vi "Set Lockin Oscillator.vi"(7 "Model":enum16{"7265", "SR830"}(ring)=enum."SR830", 9 "Amplitude":dbl=-1.0, 10 "Frequency":dbl=-1.0, 11 "VISA resource name":refnum<visa-resource-name>) -> (1 "Actual Amp":dbl, 2 "Actual Freq":dbl)   [LabVIEW 2021]
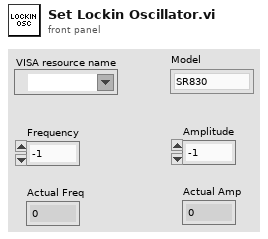
[diagram p1: front panel]
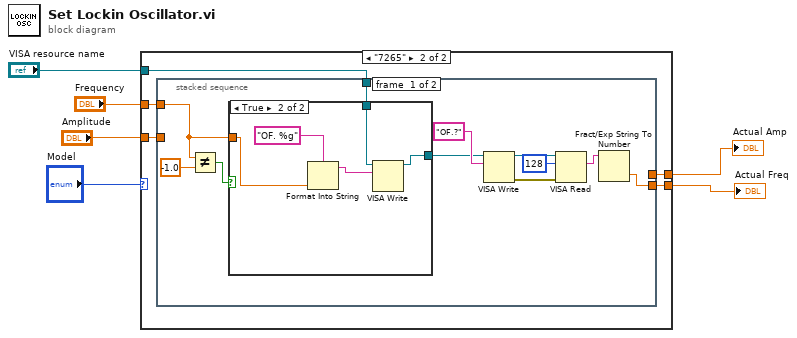
[diagram p0: block diagram]
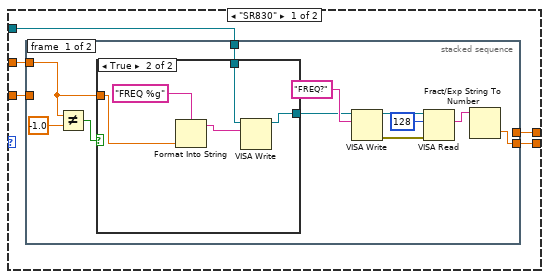
[diagram p2: hidden frame]
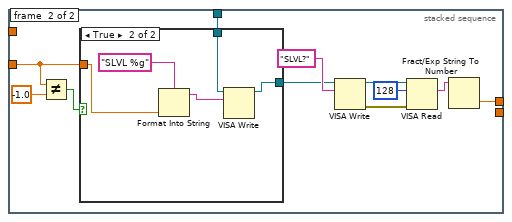
[diagram p4: hidden frame]
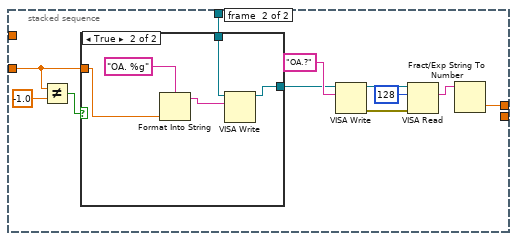
[diagram p7: hidden frame]
diagram:
  n1 = case shown="\"7265\"" "Model" {
    tunnel: "Frequency" -> [w11 w50]
    tunnel: "VISA resource name" -> [w10 w49]
    tunnel: [w9 w48] -> w3
    tunnel: "Amplitude" -> [w7 w47]
    tunnel: [w8 w46] -> w1
    frame "SR830" {
      n2 = stacked-sequence {
        tunnel: w11 -> [w20 _]
        tunnel: w10 -> [w19 w37]
        tunnel: [w12 _] -> w9
        tunnel: [_ w30] -> w8
        tunnel: w7 -> [_ w29]
        frame #0 {
          n3 = Not Equal?(x=w20, y=-1.0) -> (x != y?=w22:bool)
          n4 = case shown="True" w22 {
            tunnel: w20 -> [_ w27]
            tunnel: w19 -> [w23 w25]
            tunnel: [w23 w24] -> w13
            frame False {
            }
            frame True {
              n5 = Format Into String(format string="FREQ %g", w27) -> (resulting string=w26:string)  [unwired: 2 in, 1 out]
              n6 = VISA Write(VISA resource name=w25, write buffer=w26) -> (VISA resource name out=w24:refnum<visa-resource-name>)  [unwired: 1 in, 2 out]
            }
          }
          n7 = VISA Write(VISA resource name=w13, write buffer="FREQ?" ("format string")) -> (VISA resource name out=w17:refnum<visa-resource-name>, error out=w15:errorcluster)  [unwired: 1 in, 1 out]
          n8 = VISA Read(VISA resource name=w17, byte count=u32 128, error in (no error)=w15) -> (read buffer=w14:string)  [unwired: 3 out]
          n9 = Fract/Exp String To Number(string=w14) -> (number=w12:dbl)  [unwired: 3 in, 1 out]
        }
        frame #1 {
          n10 = Not Equal?(x=w29, y=-1.0) -> (x != y?=w39:bool)
          n11 = case shown="True" w39 {
            tunnel: w29 -> [_ w44]
            tunnel: w37 -> [w40 w42]
            tunnel: [w40 w41] -> w31
            frame False {
            }
            frame True {
              n12 = Format Into String(format string="SLVL %g", w44) -> (resulting string=w43:string)  [unwired: 2 in, 1 out]
              n13 = VISA Write(VISA resource name=w42, write buffer=w43) -> (VISA resource name out=w41:refnum<visa-resource-name>)  [unwired: 1 in, 2 out]
            }
          }
          n14 = VISA Write(VISA resource name=w31, write buffer="SLVL?" ("format string")) -> (VISA resource name out=w35:refnum<visa-resource-name>, error out=w33:errorcluster)  [unwired: 1 in, 1 out]
          n15 = VISA Read(VISA resource name=w35, byte count=u32 128, error in (no error)=w33) -> (read buffer=w32:string)  [unwired: 3 out]
          n16 = Fract/Exp String To Number(string=w32) -> (number=w30:dbl)  [unwired: 3 in, 1 out]
        }
      }
    }
    frame "7265" {
      n17 = stacked-sequence {
        tunnel: w50 -> [w59 _]
        tunnel: w49 -> [w58 w76]
        tunnel: [w51 _] -> w48
        tunnel: w47 -> [_ w69]
        tunnel: [_ w68] -> w46
        frame #0 {
          n18 = Not Equal?(x=w59, y=-1.0) -> (x != y?=w61:bool)
          n19 = case shown="True" w61 {
            tunnel: w59 -> [_ w66]
            tunnel: w58 -> [w62 w64]
            tunnel: [w62 w63] -> w52
            frame False {
            }
            frame True {
              n20 = Format Into String(format string="OF. %g", w66) -> (resulting string=w65:string)  [unwired: 2 in, 1 out]
              n21 = VISA Write(VISA resource name=w64, write buffer=w65) -> (VISA resource name out=w63:refnum<visa-resource-name>)  [unwired: 1 in, 2 out]
            }
          }
          n22 = VISA Write(VISA resource name=w52, write buffer="OF.?" ("format string")) -> (VISA resource name out=w56:refnum<visa-resource-name>, error out=w54:errorcluster)  [unwired: 1 in, 1 out]
          n23 = VISA Read(VISA resource name=w56, byte count=u32 128, error in (no error)=w54) -> (read buffer=w53:string)  [unwired: 3 out]
          n24 = Fract/Exp String To Number(string=w53) -> (number=w51:dbl)  [unwired: 3 in, 1 out]
        }
        frame #1 {
          n25 = Not Equal?(x=w69, y=-1.0) -> (x != y?=w78:bool)
          n26 = case shown="True" w78 {
            tunnel: w69 -> [_ w83]
            tunnel: w76 -> [w79 w81]
            tunnel: [w79 w80] -> w70
            frame False {
            }
            frame True {
              n27 = Format Into String(format string="OA. %g", w83) -> (resulting string=w82:string)  [unwired: 2 in, 1 out]
              n28 = VISA Write(VISA resource name=w81, write buffer=w82) -> (VISA resource name out=w80:refnum<visa-resource-name>)  [unwired: 1 in, 2 out]
            }
          }
          n29 = VISA Write(VISA resource name=w70, write buffer="OA.?" ("format string")) -> (VISA resource name out=w74:refnum<visa-resource-name>, error out=w72:errorcluster)  [unwired: 1 in, 1 out]
          n30 = VISA Read(VISA resource name=w74, byte count=u32 128, error in (no error)=w72) -> (read buffer=w71:string)  [unwired: 3 out]
          n31 = Fract/Exp String To Number(string=w71) -> (number=w68:dbl)  [unwired: 3 in, 1 out]
        }
      }
    }
  }
  "Actual Freq" <- w3
  "Actual Amp" <- w1
